vi "GT Find Subset of Operations.vi"(7 "Lambda":dbl, 8 "ESmin":u16, 9 "ECmin":u16, 10 "Earliest Start Times Array":u16[](array[numeric]), 11 "Schedule":u16[](array[numeric])) -> (2 "ES Times  SubSet Out":u16[](array[numeric]), 3 "Operation  Subset Out":u16[](array[numeric]))   [LabVIEW 2013, in "Scheduler.lvclass"]
doc: "Bu VI GT Active Scheduler icin En Erken Baslagic Zamani (ES) henuz shedule edilmemis operasyonlar icinden belirlenen minimum bitis zamanindan kucuk veya esit operasyonlari ve baslangic zamanlarini atri ayri bir alt kume olarak dondurur."
uses:
  Scheduler.lvclass
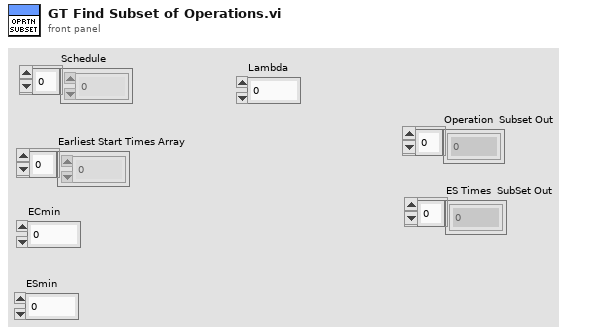
[diagram p1: front panel]
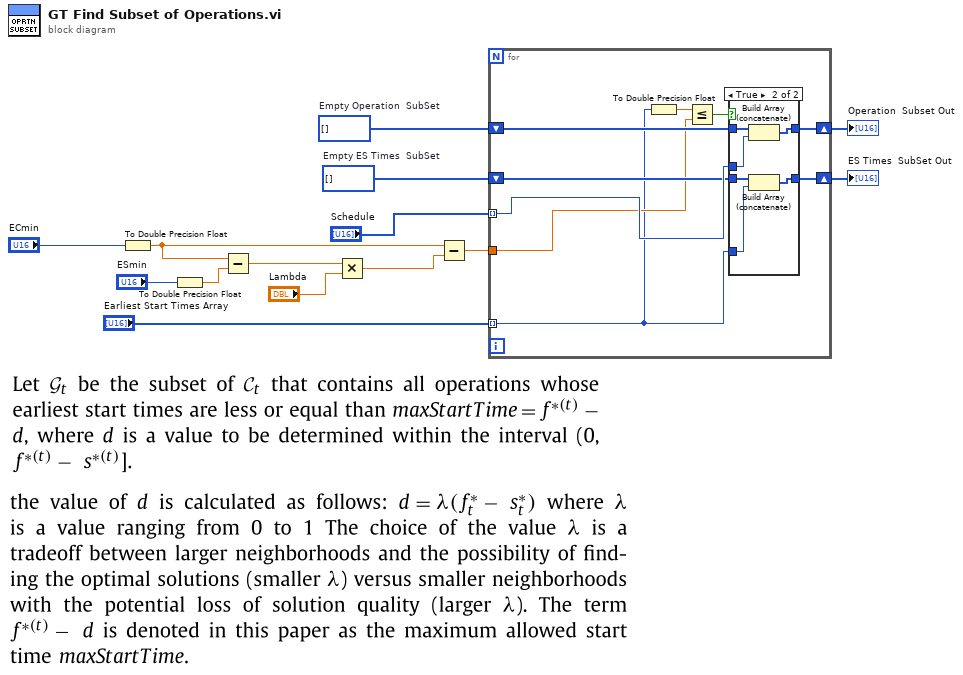
[diagram p0: block diagram]
diagram:
  w10 = u16[] []  # Empty ES Times  SubSet
  w11 = u16[] []  # Empty Operation  SubSet
  n1 = To Double Precision Float(number="ECmin") -> (double precision float=w3:dbl)
  n2 = To Double Precision Float(number="ESmin") -> (double precision float=w7:dbl)
  n3 = Subtract(x=w3, y=w7) -> (x-y=w4:dbl)
  n4 = Multiply(x=w4, y="Lambda") -> (x*y=w2:dbl)
  n5 = Subtract(x=w3, y=w2) -> (x-y=w1:dbl)
  n6 = for {
    tunnel: "Schedule" -> [w21] mode=indexing
    tunnel: "Earliest Start Times Array" -> [w16] mode=indexing
    shift-right: [w20] -> w12
    shift-left: w11 -> [w23]
    shift-right: [w18] -> w9
    shift-left: w10 -> [w19]
    tunnel: w1 -> [w17]
    n7 = To Double Precision Float(number=w16) -> (double precision float=w15:dbl)
    n8 = Less Or Equal?(x=w15, y=w17) -> (x <= y?=w22:bool)
    n9 = case shown="True" w22 {
      tunnel: w23 -> [w25 w31]
      tunnel: w21 -> [_ w30]
      tunnel: [w25 w29] -> w20
      tunnel: w19 -> [w24 w28]
      tunnel: [w24 w26] -> w18
      tunnel: w16 -> [_ w27]
      frame False {
      }
      frame True {
        n10 = Build Array (concatenate)(w31, w30) -> (w29:u16[])
        n11 = Build Array (concatenate)(w28, w27) -> (w26:u16[])
      }
    }
  }
  "Operation  Subset Out" <- w12
  "ES Times  SubSet Out" <- w9
